vi "SetPoint.vi"(8 "error in (no error)":errorcluster, 10 "Point":refnum<class "Point.lvclass">, 11 "Circle in":refnum<class "Circle.lvclass">) -> (0 "error out":errorcluster, 3 "Circle out":refnum<class "Circle.lvclass">)   [LabVIEW 2021, in "Picture2D.lvlib" / "Circle.lvclass"]
uses:
  Circle.lvclass
  Shape/Shape.lvclass
  Point/Point.lvclass
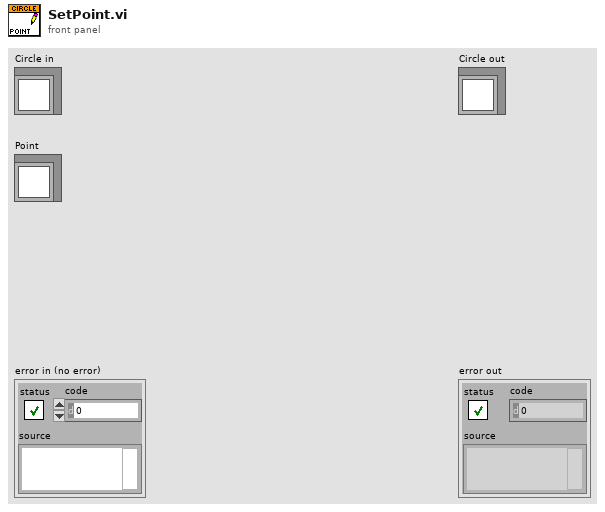
[diagram p1: front panel]
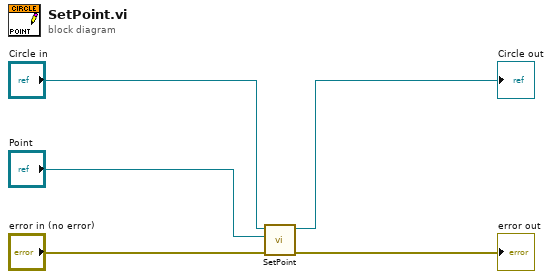
[diagram p0: block diagram]
diagram:
  n1 = call-parent "SetPoint.vi"("error in (no error)"="error in (no error)", "Point"="Point", "Picture2D in"="Circle in") -> ("error out"=→"error out":errorcluster, "Picture2D out"=→"Circle out":refnum<class "Circle.lvclass">)  [unwired: 7 in]
